vi "Robot Global Data.vi"() -> ()   [LabVIEW 2013]
doc: "This global VI can contain as many global variables as you need. Place a control on the panel, give it a good name. To read or write to it from a VI, drag the icon to the diagram of that VI. You can also drag from the project. Click on the node to change which global you access. You shouldn't have multiple locations writing to a global or it will cause a race-condition."
uses:
  <vilib>/Rock Robotics/WPI/Camera/WPI_CameraImageSize.ctl
  <vilib>/Rock Robotics/WPI/DriverStation/WPI_DriverStationRobotMode2.ctl
panel:
  in  "Cranking In":bool
  in  "Three-Fourths of a Second Ago":dbl=100.0
  in  "Crankback Auto?":bool
  in  "Auto Stop Reference":bool
  in  "Auto Arms Close":bool
  in  "Auto Arms Open":bool
  in  "Driver Arms":bool
  in  "Driver Turret":bool
  in  "Goal is Hot":bool
  in  "Firing Arm Release":bool
  in  "Primed to Fire":bool
  in  "Locking":bool
  in  "Ready to Lock":bool
  in  "Locked":bool
  in  "Wingman Joystick":T1
  in  "Shooter Locked":bool
  in  "Auto Spin":bool
  in  "Arm Closing":bool
  in  "Turret Stop":bool
  in  "Spin Roller":bool
  in  "Turret Angle":dbl
  in  "Turret Moving Down":bool
  in  "Turret Moving Up":bool
  in  "Drive to Position":T2
  in  "Position":cluster{"X":dbl, "Y":dbl, "Angle":dbl}={"X"=0.0, "Y"=144.0, "Angle"=180.0}
  in  "Search Mode Activated":bool
  in  "Search Mode":bool
  in  "End of Match release":bool
  in  "Automatic Drive Right":dbl
  in  "Shoot":bool
  in  "Auto Target Rotate Speed":dbl
  in  "Auto Target":bool
  in  "Automatic Drive Left":dbl
  in  "Left Joystick":T1
  in  "Right Joystick":T1
  in  "Auto Drive?":bool
  in  "Vision Testing Drive":dbl
  in  "Robot Mode":T3
  in  "LED toggle rate (ms)":u32=20
  in  "image size":T4=enum."320x240"
  in  "Enable Vision":bool
  # "e"
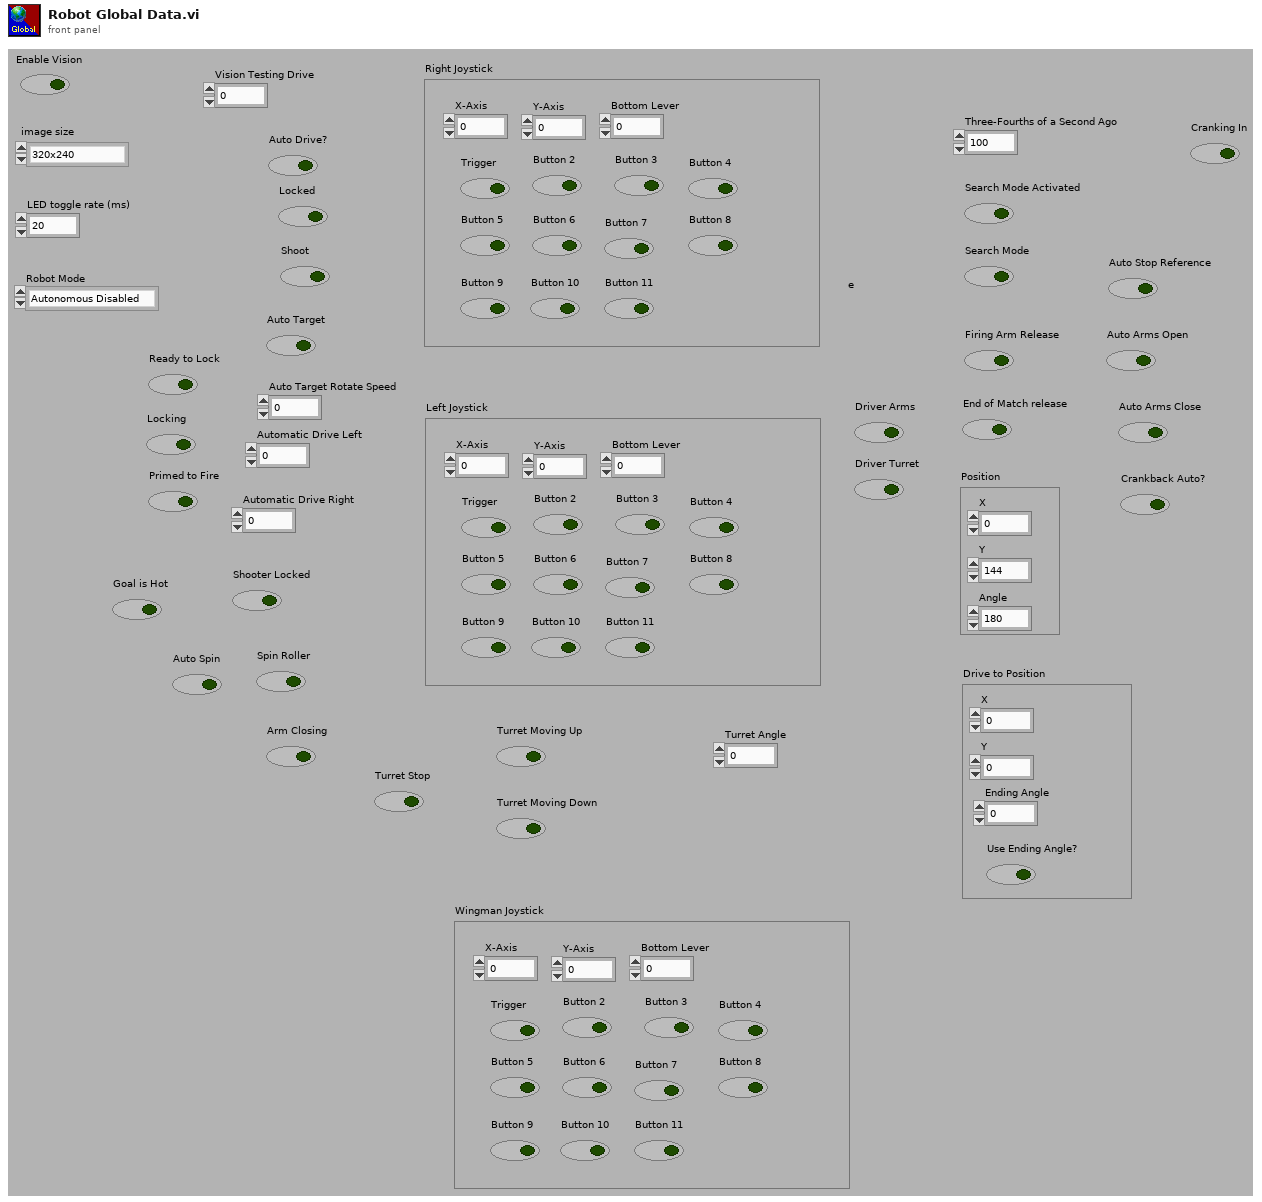
[diagram p1: front panel]
types:
  T1 = cluster{"X-Axis":dbl, "Y-Axis":dbl, "Bottom Lever":dbl, "Trigger":bool, "Button 2":bool, "Button 3":bool, "Button 4":bool, "Button 5":bool, "Button 6":bool, "Button 7":bool, "Button 8":bool, "Button 9":bool, "Button 10":bool, "Button 11":bool}
  T2 = cluster{"X":dbl, "Y":dbl, "Ending Angle":dbl, "Use Ending Angle?":bool}
  T3 = typedef "WPI_DriverStationRobotMode2.ctl" = enum16{"Autonomous Disabled", "Autonomous Enabled", "Teleop Disabled", "Teleop Enabled", "Timeout", "Finish", "Test Disabled", "Test Enabled"}
  T4 = typedef "WPI_CameraImageSize.ctl" = enum16{"640x480", "320x240", "160x120"}
diagram:
